vi "Protocol.Network.Command Handler.vi"(8 "error in (no error)":errorcluster, 11 "J1939 Main Configuration":T1) -> (0 "error out":errorcluster)   [LabVIEW 2015, in "J1939 Addon Engine.lvlib"]
uses:
  J1939 Addon Engine.lvlib
  Types/Protocol.Configuration.ctl
  <vilib>/NI/NIVS Addon Network Comm/Engine/VeriStand Comm.lvclass
  <vilib>/NI/NIVS Inline Async API/_VS Inline Async API/Process/Process.lvclass
  Types/Protocol.Refs.ctl
  Shared/J1939 Utilities/Types/CAN Outgoing Message Cluster.ctl
  Types/Protocol.RQST Lookup Table Reference.ctl
  Types/Protocol.Address Table Reference.ctl
  Types/Protocol.XNET Settings.ctl
  <vilib>/NI/NIVS Inline Async API/_Data Access Engine/Data Access Engine/Types/Read.DVR.ctl
  <vilib>/NI/NIVS Inline Async API/_Data Access Engine/Access Type Classes/Read/Read.lvclass
  <vilib>/NI/NIVS Inline Async API/_Data Access Engine/Data Access Engine/Types/Write.DVR.ctl
  <vilib>/NI/NIVS Inline Async API/_Data Access Engine/Access Type Classes/Write/Write.lvclass
  Types/CounterAndProtectionFrames.ctl
  SubModules/Frame Protection Support/Source/Engine/Types/RT Frame Settings.ctl
  SubModules/Frame Protection Support/Source/Shared/Types/Exported Frame Type.ctl
  SubModules/Frame Protection Support/Source/Engine/Types/RT Protection Configuration.ctl
  SubModules/Frame Protection Support/Source/Shared/Types/Protection Type.ctl
  SubModules/Frame Protection Support/Source/Shared/Types/XNET Signal Configuration.ctl
  SubModules/Frame Protection Support/Source/Shared/Types/Exported Counter Settings.ctl
  SubModules/Frame Protection Support/Source/Shared/Types/Exported Event Trigger Type.ctl
  <vilib>/NI/NIVS Addon Network Comm/Engine/VeriStand Comm.lvclass/VeriStand Comm.ctl
  Shared/Types/Request Message.ctl
  Types/Protocol.Address Lookup Table Action.ctl
  <vilib>/NI/NIVS Inline Async API/_VS Inline Async API/Process/Process.lvclass/Process.ctl
  Shared/J1939 Utilities/SubVIs/Convert CAN Arb ID to J1939 ID.vi
  <vilib>/NI/NIVS Inline Async API/_VS Inline Async API/Error Handling Process/SubVIs/Error.ConvertArray.vi
  <vilib>/NI/AMC/Read Next Message.vi
  <vilib>/NI/Tools/Keyed Array/Index.vi
  Shared/J1939 Utilities/Common Messages.vi
  Shared/J1939 Utilities/SubVIs/Request.vi
  Protocol.RQST Lookup Table Act.vi
  <vilib>/NI/AMC/Send Local Message.vi
  <vilib>/NI/AMC/Read Termination Message.vi
  <vilib>/NI/Tools/Keyed Array/Map String.vi
  Shared/J1939 Utilities/SubVIs/Convert J1939 ID to CAN Arb ID.vi
  <vilib>/NI/AMC/Create Single Message.vi
  <vilib>/NI/AMC/Update Message Routing Info.vi
  <vilib>/NI/Tools/String/Get Case Matching.vi
  <vilib>/NI/AMC/Send Message.vi
  Protocol.Address Lookup Table.vi
  <vilib>/xnet/xnet.llb/XNET Read (State CAN Comm).vi
  Protocol.RQST Lookup Table.vi
  <vilib>/NI/AMC/Globals.vi
  <vilib>/NI/NIVS Addon Network Comm/Shared/Comm Constants.vi
  Shared/J1939 Addon Shared.lvlib
  Shared/J1939 Utilities/J1939 Utilities.lvlib
  <vilib>/NI VeriStand/Custom Device Tools/Custom Device Utility Library/Custom Device Utility Library.lvlib
  <vilib>/NI/NIVS Inline Async API/_Data Access Engine/Data Access Engine/Data Access Engine.lvclass
  SubModules/Frame Protection Support/Source/Engine/Protection and Counter Support Engine.lvlib
  SubModules/Frame Protection Support/Source/Shared/Protection and Counter Support Shared.lvlib
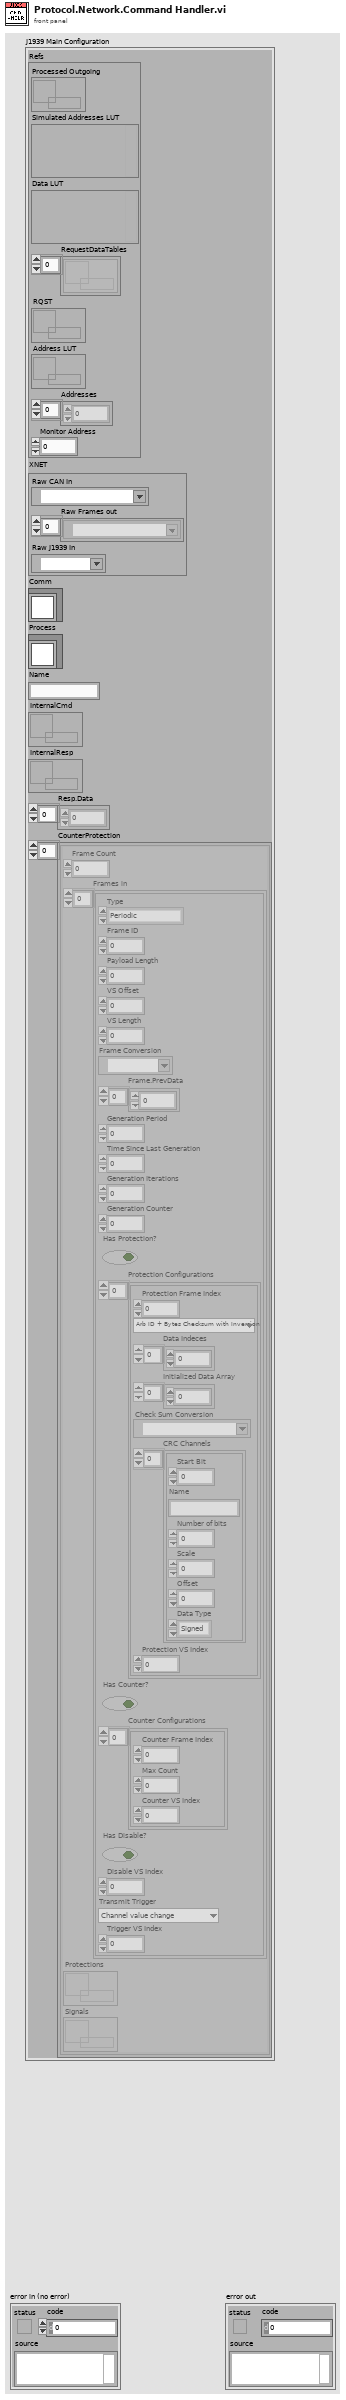
[diagram p1: front panel]
types:
  T1 = typedef "J1939 Addon Engine.lvlib/Protocol.Configuration.ctl" = cluster{"Refs":T2, "XNET":T5, "Comm":refnum<class "VeriStand Comm.lvclass">, "Process":refnum<class "Process.lvclass">, "Name":string, "InternalCmd":T6, "InternalResp":T7, "Resp.Data":dbl[], "CounterProtection":T8[]}
  T2 = typedef "J1939 Addon Engine.lvlib/Protocol.Refs.ctl" = cluster{"Processed Outgoing":refnum<queue>, "Simulated Addresses LUT":variant, "Data LUT":variant, "RequestDataTables":refnum<k33>[], "RQST":T3, "Address LUT":T4, "Addresses":u8[], "Monitor Address":u8}
  T3 = typedef "J1939 Addon Engine.lvlib/Protocol.RQST Lookup Table Reference.ctl" = refnum<data-value>
  T4 = typedef "J1939 Addon Engine.lvlib/Protocol.Address Table Reference.ctl" = refnum<data-value>
  T5 = typedef "J1939 Addon Engine.lvlib/Protocol.XNET Settings.ctl" = cluster{"Raw CAN In":refnum<k21>, "Raw Frames out":refnum<k21>[], "Raw J1939 In":refnum<k21>}
  T6 = typedef "Data Access Engine.lvlib/Data Access Engine.lvclass/Read.DVR.ctl" = refnum<data-value>
  T7 = typedef "Data Access Engine.lvlib/Data Access Engine.lvclass/Write.DVR.ctl" = refnum<data-value>
  T8 = typedef "J1939 Addon Engine.lvlib/CounterAndProtectionFrames.ctl" = cluster{"Frame Count":i32, "Frames in":T9[], "Protections":T7, "Signals":T6}
  T9 = typedef "Protection and Counter Support Engine.lvlib/RT Frame Settings.ctl" = cluster{"Type":T10, "Frame ID":u32, "Payload Length":u32, "VS Offset":i32, "VS Length":i32, "Frame Conversion":refnum<k21>, "Frame.PrevData":dbl[], "Generation Period":u32, "Time Since Last Generation":u32, "Generation Iterations":u32, "Generation Counter":u32, "Has Protection?":bool, "Protection Configurations":T11[], "Has Counter?":bool, "Counter Configurations":T14[], "Has Disable?":bool, "Disable VS Index":i32, "Transmit Trigger":T15, "Trigger VS Index":i32}
  T10 = typedef "Protection and Counter Support Shared.lvlib/Exported Frame Type.ctl" = enum16{"Periodic", "Event", "Periodic/Event"}
  T11 = typedef "Protection and Counter Support Engine.lvlib/RT Protection Configuration.ctl" = cluster{"Protection Frame Index":i32, "Protection Type":T12, "Data Indeces":i32[], "Initialized Data Array":dbl[], "Check Sum Conversion":refnum<k21>, "CRC Channels":T13[], "Protection VS Index":i32}
  T12 = typedef "Protection and Counter Support Shared.lvlib/Protection Type.ctl" = enum16{"Arb ID + Bytes Checksum with Inversion", "Arb ID + Bytes CRC with Inversion", "Reversed Raw Signal Checksum with Inversion"}
  T13 = typedef "Protection and Counter Support Shared.lvlib/XNET Signal Configuration.ctl" = cluster{"Start Bit":i32, "Name":string, "Number of bits":i32, "Scale":dbl, "Offset":dbl, "Data Type":u32}
  T14 = typedef "Protection and Counter Support Shared.lvlib/Exported Counter Settings.ctl" = cluster{"Counter Frame Index":i32, "Max Count":dbl, "Counter VS Index":i32}
  T15 = typedef "Protection and Counter Support Shared.lvlib/Exported Event Trigger Type.ctl" = enum16{"Channel value change", "Trigger channel (not zero)", "Channel value change or trigger channel (not zero)", "Trigger channel (any value change)", "Channel value change or trigger channel (any value change)"}
  T16 = typedef "J1939 Addon Shared.lvlib/Request Message.ctl" = cluster{"PGN":u32, "DA":u8, "Ignore Response":bool}
  T17 = typedef "J1939 Addon Shared.lvlib/J1939 Utilities.lvlib/CAN Outgoing Message Cluster.ctl" = cluster{"Identifier":u32, "Data":u8[]}
  T18 = typedef "J1939 Addon Engine.lvlib/Protocol.Address Lookup Table Action.ctl" = enum16{"Initialize", "Add", "Get", "Remove", "Get All"}
  T19 = typedef "NI VeriStand Addon Network Comm.lvlib/VeriStand Comm.lvclass/Response Information.ctl" = cluster{"response name":string, "responseQ":string}
  T20 = typedef "XNET Frame CAN.ctl" = cluster{"timestamp":timestamp, "payload":u8[], "identifier":u32, "type":T21, "extended?":bool, "echo?":bool}
  T21 = typedef "XNET Frame Type CAN.ctl" = u8
  T22 = typedef "XNET CAN Comm.ctl" = cluster{"fault code":i32, "fault?":bool, "communication state":T23, "last error":T24, "receive error counter":u8, "transmit error counter":u8, "transceiver error?":bool, "sleep?":bool}
  T23 = typedef "XNET CAN Comm State.ctl" = u8
  T24 = typedef "XNET CAN Last Err.ctl" = u8
  T25 = typedef "J1939 Addon Shared.lvlib/Address Lookup Table Data.ctl" = cluster{"Name":u8[], "Address":u8}
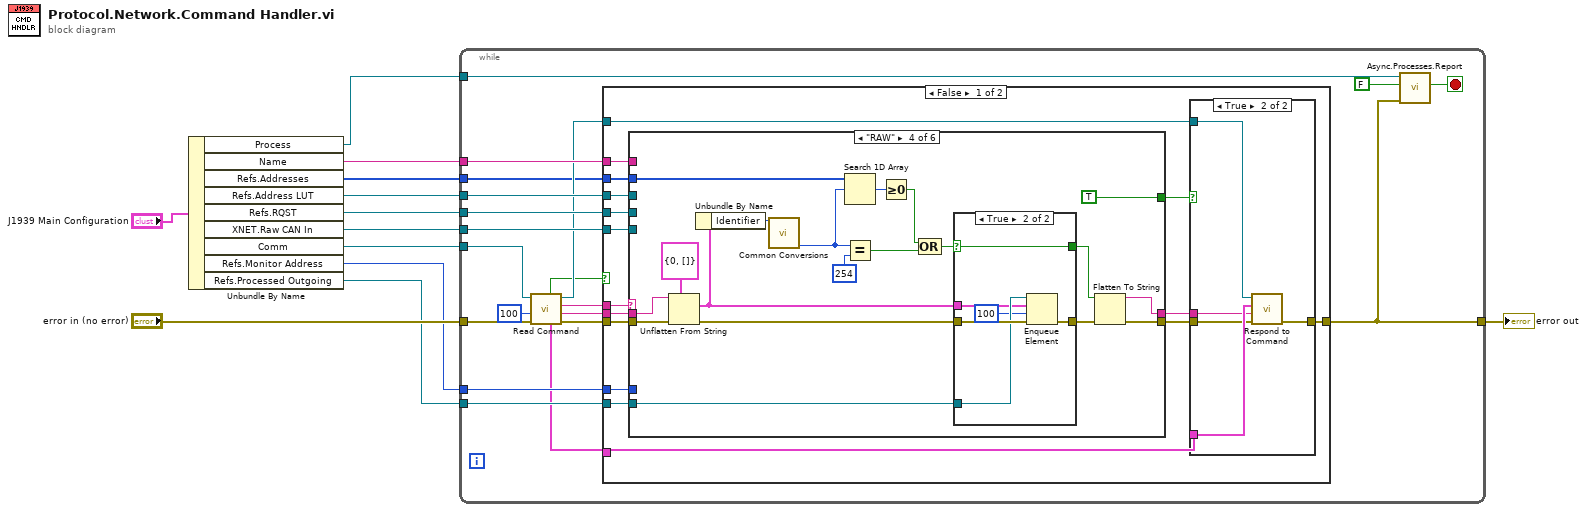
[diagram p0: block diagram]
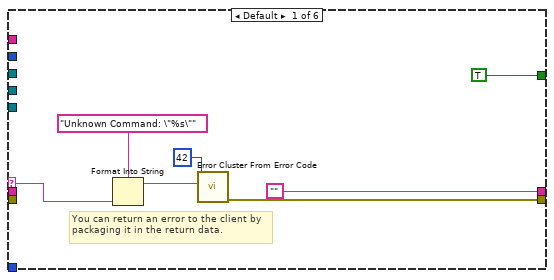
[diagram p3: hidden frame]
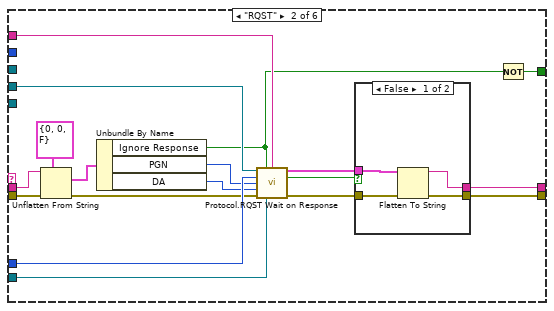
[diagram p4: hidden frame]
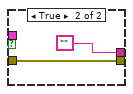
[diagram p5: hidden frame]
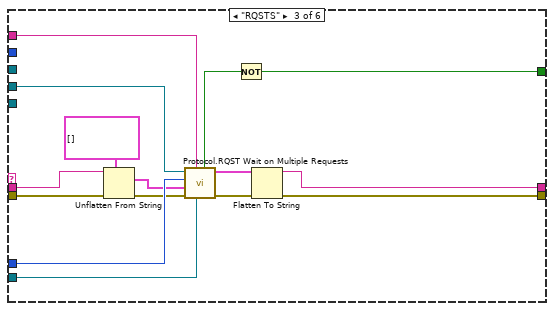
[diagram p6: hidden frame]
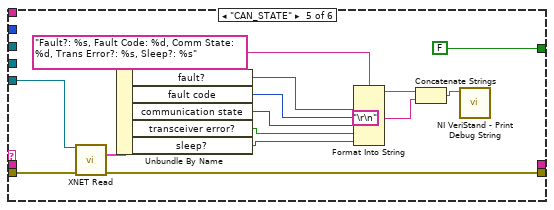
[diagram p8: hidden frame]
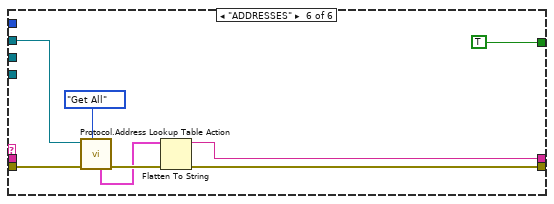
[diagram p9: hidden frame]
diagram:
  n1 = Unbundle By Name("J1939 Main Configuration") -> ("Process"=w3:refnum<class "Process.lvclass">, "Name"=w4:string, "Refs.Addresses"=w1:u8[], "Refs.Address LUT"=w5:T4, "Refs.RQST"=w6:T3, "XNET.Raw CAN In"=w7:refnum<k21>, "Comm"=w8:refnum<class "VeriStand Comm.lvclass">, "Refs.Monitor Address"=w9:u8, "Refs.Processed Outgoing"=w10:refnum<queue>)
  n2 = while {
    tunnel: "error in (no error)" -> [w29]
    tunnel: [w21] -> w11
    tunnel: w3 -> [w31]
    tunnel: w8 -> [w28]
    tunnel: w4 -> [w27]
    tunnel: w7 -> [w26]
    tunnel: w10 -> [w25]
    tunnel: w9 -> [w24]
    tunnel: w6 -> [w23]
    tunnel: w5 -> [w22]
    tunnel: w1 -> [w13]
    stop <- w32 stop-if-true
    n3 = call <vilib>:"Read Command.vi"("error in (no error)"=w29, "timeout (100 ms)"=100, "VeriStand Comm in"=w28) -> ("error out"=w19:errorcluster, "message value"=w17:string, "message name"=w18:string, "VeriStand Comm out"=w15:refnum<class "VeriStand Comm.lvclass">, "ResponseInfo"=w16:T19, "timed out?"=w14:bool)  [unwired: 3 in]
    n4 = case shown="False" w14 {
      tunnel: w27 -> [w48 _]
      tunnel: w26 -> [w47 _]
      tunnel: w25 -> [w46 _]
      tunnel: w24 -> [w45 _]
      tunnel: w23 -> [w44 _]
      tunnel: w22 -> [w43 _]
      tunnel: [w42 w150] -> w21
      tunnel: w19 -> [w41 w150]
      tunnel: w18 -> [w40 _]
      tunnel: w17 -> [w39 _]
      tunnel: w16 -> [w38 _]
      tunnel: w15 -> [w37 _]
      tunnel: w13 -> [w33 _]
      frame False {
        n5 = case shown="\"RAW\"" w40 {
          selector: w40 -> [w57 _ _ _ _ _]
          tunnel: w39 -> [_ w66 w86 w118 _ _]
          tunnel: [w58 w78 w87 w102 w139 w143] -> w35
          tunnel: ["" ("data string") w75 w100 w101 _ w144] -> w36
          tunnel: w46 -> [_ w73 w98 w116 _ _]
          tunnel: w41 -> [_ w72 w90 w119 w141 w148]
          tunnel: w44 -> [_ w65 w97 _ _ _]
          tunnel: w45 -> [_ w79 w96 _ _ _]
          tunnel: w43 -> [_ _ _ _ _ w147]
          tunnel: w48 -> [_ w64 w93 _ _ _]
          tunnel: w47 -> [_ _ _ _ w140 _]
          tunnel: [TRUE w62 w91 TRUE FALSE TRUE] -> w34
          tunnel: w33 -> [_ _ _ w111 _ _]
          frame Default {
            # "You can return an error to the client by packaging it in the return data."
            n6 = Format Into String(format string="Unknown Command: \"%s\"", w57) -> (resulting string=w59:string)  [unwired: 2 in, 1 out]
            n7 = call <vilib>:"Error Cluster From Error Code.vi"("error message (\"\")"=w59, "error code (0)"=42) -> ("error out"=w58:errorcluster)  [unwired: 7 in]
          }
          frame "RQST" {
            n8 = Unflatten From String(type=T16 {"PGN"=0, "DA"=0, "Ignore Response"=FALSE} ("Cluster"), binary string=w66, error in (no error)=w72) -> (value=w69:T16, error out=w71:errorcluster)  [unwired: 2 in, 1 out]
            n9 = Unbundle By Name(w69) -> ("Ignore Response"=w63:bool, "PGN"=w68:u32, "DA"=w67:u8)
            n10 = call "Protocol.RQST Wait on Response.vi"("ref in"=w65, "Ignore Response"=w63, "Name"=w64, "Source Address"=w79, "PGN"=w68, "DA"=w67, "error in (no error)"=w71, "Processed Outgoing"=w73) -> ("element"=w74:T20, "timed out?"=w76:bool, "error out"=w77:errorcluster)  [unwired: 4 in, 1 out]
            n11 = case shown="False" w76 {
              tunnel: [w81 w85] -> w78
              tunnel: w77 -> [w82 w85]
              tunnel: [w80 ""] -> w75
              tunnel: w74 -> [w83 _]
              frame False {
                n12 = Flatten To String(anything=w83, error in (no error)=w82) -> (data string=w80:string, error out=w81:errorcluster)  [unwired: 2 in, 1 out]
              }
              frame True {
              }
            }
            n13 = Not(x=w63) -> (.not. x?=w62:bool)
          }
          frame "RQSTS" {
            n14 = Unflatten From String(type=T16[] [], binary string=w86, error in (no error)=w90) -> (value=w95:T16[], error out=w89:errorcluster)  [unwired: 2 in, 1 out]
            n15 = call "Protocol.RQST Wait on Multiple Requests.vi"("Processed Outgoing"=w98, "Name"=w93, "error in (no error)"=w89, "value"=w95, "Source Address"=w96, "ref in"=w97) -> ("error out"=w88:errorcluster, "Elements"=w94:T20[], "Ignore Response?"=w92:bool)  [unwired: 1 in, 2 out]
            n16 = Not(x=w92) -> (.not. x?=w91:bool)
            n17 = Flatten To String(anything=w94, error in (no error)=w88) -> (data string=w100:string, error out=w87:errorcluster)  [unwired: 2 in, 1 out]
          }
          frame "RAW" {
            n18 = Unflatten From String(type=T17 {"Identifier"=0, "Data"=[]} ("Data to Send"), binary string=w118, error in (no error)=w119) -> (value=w114:T17, error out=w105:errorcluster)  [unwired: 2 in, 1 out]
            n19 = Unbundle By Name(w114) -> ("Identifier"=w113:u32)
            n20 = call-poly "Common Conversions.vi"("Arb ID"=w113) -> ("Source Address"=w110:u8)  [unwired: 11 in, 3 out]
            n21 = Search 1D Array(1D array=w111, element=w110) -> (index of element=w109:i32)  [unwired: 1 in]
            n22 = Equal?(x=w110, y=u8 254) -> (x = y?=w107:bool)
            n23 = Greater Or Equal To 0?(x=w109) -> (x >= 0?=w108:bool)
            n24 = Compound Arithmetic op=OR(w108, w107) -> (w106:bool)
            n25 = case shown="True" w106 {
              selector: w106 -> [w120 w122]
              tunnel: w105 -> [w121 w127]
              tunnel: w116 -> [_ w126]
              tunnel: [w121 w124] -> w103
              tunnel: w114 -> [_ w123]
              tunnel: [w120 w122] -> w104
              frame False {
              }
              frame True {
                n26 = Enqueue Element(queue=w126, element=w123, timeout in ms (-1)=100, error in (no error)=w127) -> (error out=w124:errorcluster)  [unwired: 2 out]
              }
            }
            n27 = Flatten To String(anything=w104, error in (no error)=w103) -> (data string=w101:string, error out=w102:errorcluster)  [unwired: 2 in, 1 out]
          }
          frame "CAN_STATE" {
            n28 = call-poly <vilib>:"XNET Read.vi"("session in"=w140, "error in (no error)"=w141) -> ("CAN comm"=w138:T22, "error out"=w139:errorcluster)  [unwired: 11 in, 1 out]
            n29 = Unbundle By Name(w138) -> ("fault?"=w137:bool, "fault code"=w136:i32, "communication state"=w135:T23, "transceiver error?"=w134:bool, "sleep?"=w133:bool)
            n30 = Format Into String(format string="Fault?: %s, Fault Code: %d, Comm State: %d, Trans Error?: %s, Sleep?: %s", w137, w136, w135, w134, w133) -> (resulting string=w132:string)  [unwired: 2 in, 1 out]
            n31 = Concatenate Strings(w132, "\r\n") -> (w130:string)
            n32 = call <vilib>:"NI VeriStand - Print Debug String.vi"("Message"=w130) -> ()  [unwired: 10 in, 1 out]
          }
          frame "ADDRESSES" {
            n33 = call "Protocol.Address Lookup Table Action.vi"("Action"=Protocol.Address_Lookup_Table_Action."Get All", "error in (no error)"=w148, "ref in"=w147) -> ("error out"=w146:errorcluster, "All Data"=w145:T25[])  [unwired: 5 in, 2 out]
            n34 = Flatten To String(anything=w145, error in (no error)=w146) -> (data string=w144:string, error out=w143:errorcluster)  [unwired: 2 in, 1 out]
          }
        }
        n35 = case shown="True" w34 {
          tunnel: [w49 w54] -> w42
          tunnel: w38 -> [_ w53]
          tunnel: w37 -> [_ w52]
          tunnel: w36 -> [_ w51]
          tunnel: w35 -> [w49 w50]
          frame False {
          }
          frame True {
            n36 = call <vilib>:"Respond to Command.vi"("error in (no error)"=w50, "message value"=w51, "ResponseInfo"=w53, "VeriStand Comm in"=w52) -> ("error out"=w54:errorcluster)  [unwired: 5 in, 2 out]
          }
        }
      }
      frame True {
      }
    }
    n37 = call <vilib>:"Async.Processes.Report.vi"("Error"=w21, "Stop Async on Error?"=FALSE ("Stop on Error?"), "Process in"=w31) -> ("Stop"=w32:bool)  [unwired: 7 in, 1 out]
  }
  "error out" <- w11
